vi "Euclidean distance.vi"(2 "Position":i32[](array[numeric]), 3 "Position 2":i32[](array[numeric])) -> (6 "Distance":dbl)   [LabVIEW 2013]
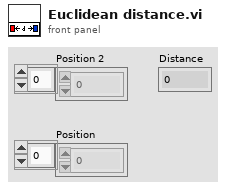
[diagram p1: front panel]
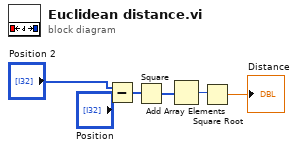
[diagram p0: block diagram]
diagram:
  n1 = Subtract(x="Position 2", y="Position") -> (x-y=w3:i32[])
  n2 = Square(x=w3) -> (x^2=w4:i32[])
  n3 = Add Array Elements(numeric array=w4) -> (sum=w5:i32)
  n4 = Square Root(x=w5) -> (sqrt(x)=→"Distance":dbl)
